vi "Frog ear specs.vi"(0 "ear folder path":path=path "/AJH L1.226B Q800/LabVIEW 3.0.1/Data/MEB/94/09/06.01/Ear 1") -> ()   [LabVIEW 2010]
panel:
  in  "time BPN' thaw":string="Time of BPN' thawing: XX"
  in  "OM removal":string="Ease of OM removal: XX"
  in  "Rating criterion":string="NOTE: Answer relative questions with a 1-10 scale (1 worst case; 10 ideal)"
  in  "mass":string="Mass (g): XX - XX"
  in  "Length (mm)":string="Length (mm): XX (mouth tip to extended leg) - XX"
  in  "Sex":string="Sex: XX"
  in  "Other comments about preparation:":string="Other comments about preparation: none"
  in  "Other comments about organ mounting:":string="Other comments about organ mounting: none"
  in  "Other comments about BPN'ing:":string="Other comments about BPN'ing: none"
  in  "Other comments about organ attainment:":string="Other comments about organ attainment: none"
  in  "Seeming approachability to kcbs:":string="Seeming approachability to kcbs: XX"
  in  "Perpendicularity of hb stereocilia:":string="Perpendicularity of hb stereocilia:  XX"
  in  "Amount of goo & crystals around hbs:":string="Amount of goo & crystals around hbs: XX"
  in  "Hair bundles' general condition:":string="Hair bundles' general condition: XX"
  in  "Amount of any further NSE desintegration:":string="Amount of any further NSE desintegration: XX"
  in  "Closeness of nerve cut to macula:":string="Closeness of nerve cut to macula: XX"
  in  "Flatness of macula as judged from dissection scope:":string="Macular flatness: XX"
  in  "Amount of sticking of organ to Pasteur pipette while transfereing organ from BPN' dish to solution dish to experimental chamber:":string="Amount of sticking of organ to Pasteur pipette while transfereing organ from BPN' dish to solution dish to chamber: XX"
  in  "# pins used to mount organ:":string="# pins used to mount organ: XX"
  in  "Amount of NSE desintegrationduring BPN'ing:":string="Amount of NSE degradation during BPN'ing: XX"
  in  "Organ BPN'ing facing:":string="Organ BPN'ing facing: XX"
  in  "Amount of sticking of organ to Pasteur pipette while transfereing organ to BPN' dish:":string="Amount of sticking of organ to Pasteur pipette while transfereing organ to BPN' dish: XX"
  in  "OM peeling?":string="Portion of OM peeled away: XX"
  in  "Crystals over OM?":string="Amount of leftover crystals atop OM: XX"
  in  "Leftover NSE goo?":string="Amount of leftover NSE goo: XX"
  in  "Any mechanical trauma to ear during organ dissection from inner ear?":string="Mechanical trauma to ear during organ dissection from inner ear: XX"
  in  "Goo removal easy?":string="Ease of goo removal: XX"
  in  "Inner ear removal from frog head through a meniscus?":string="Inner ear removal from frog head through a meniscus (T/F): XX"
  in  "Mechanical trauma to organ during inner ear dissection from animal:":string="Mechanical trauma to organ during inner ear dissection from animal: XX"
  in  "Saline oxygenation time (min)":string="Solution oxygenation time: XX"
  in  "OK; save & end":bool
  in  "BPN' time (min)":string="BPN' time (min): XX"
  in  "[BPN'] (mg/ml)":string="[BPN'] (mg/ml): XX"
  in  "Dissection solution":string="Dissection solution: Standard saline"
  in  "Organ":string="Organ: Sacculus"
  in  "Animal species":string="Species: Rana catesbeiana"
  in  "Animal death time":string="Time of death: XX"
  # "HARD SPECS:"
  # "SOLUTIONS:"
  # "ORGAN ATTAINMENT:"
  # "BPN'ing:"
  # "ORGAN MOUNTING:"
  # "CELLULAR (as judged under experimental scope):"
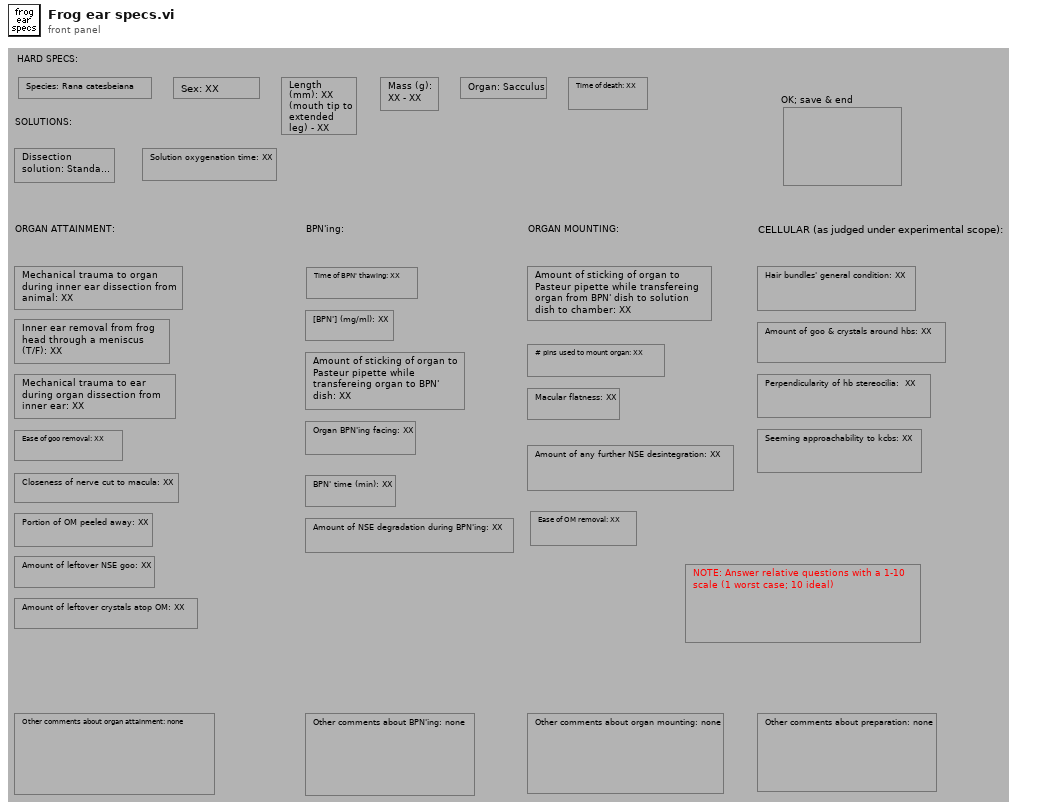
[diagram p1: front panel]
types:
  T1 = cluster{i32, i32, i32, i32, i32, i32, i32, i32, i32}
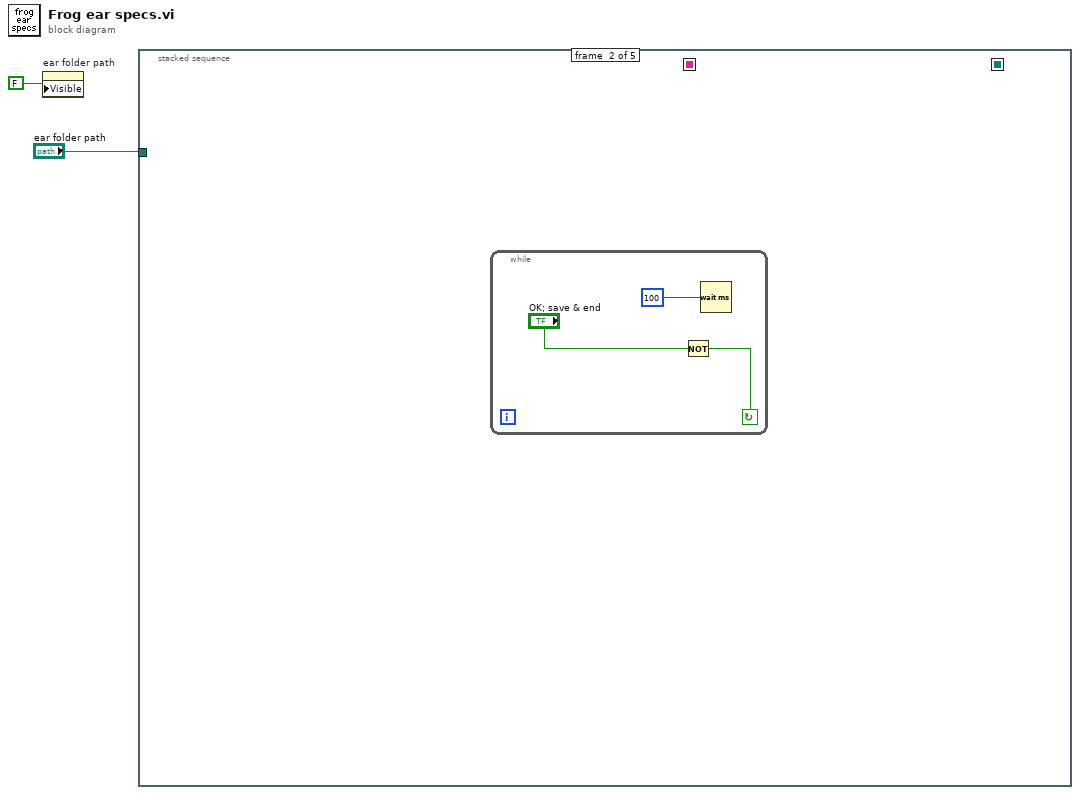
[diagram p0: block diagram]
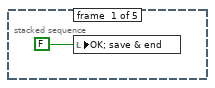
[diagram p2: hidden frame]
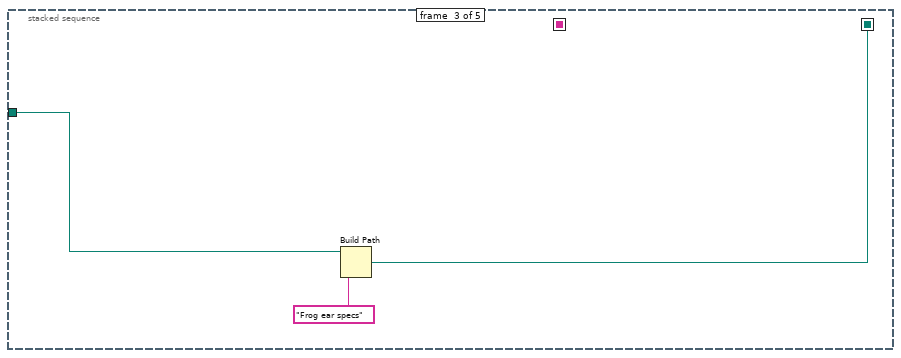
[diagram p3: hidden frame]
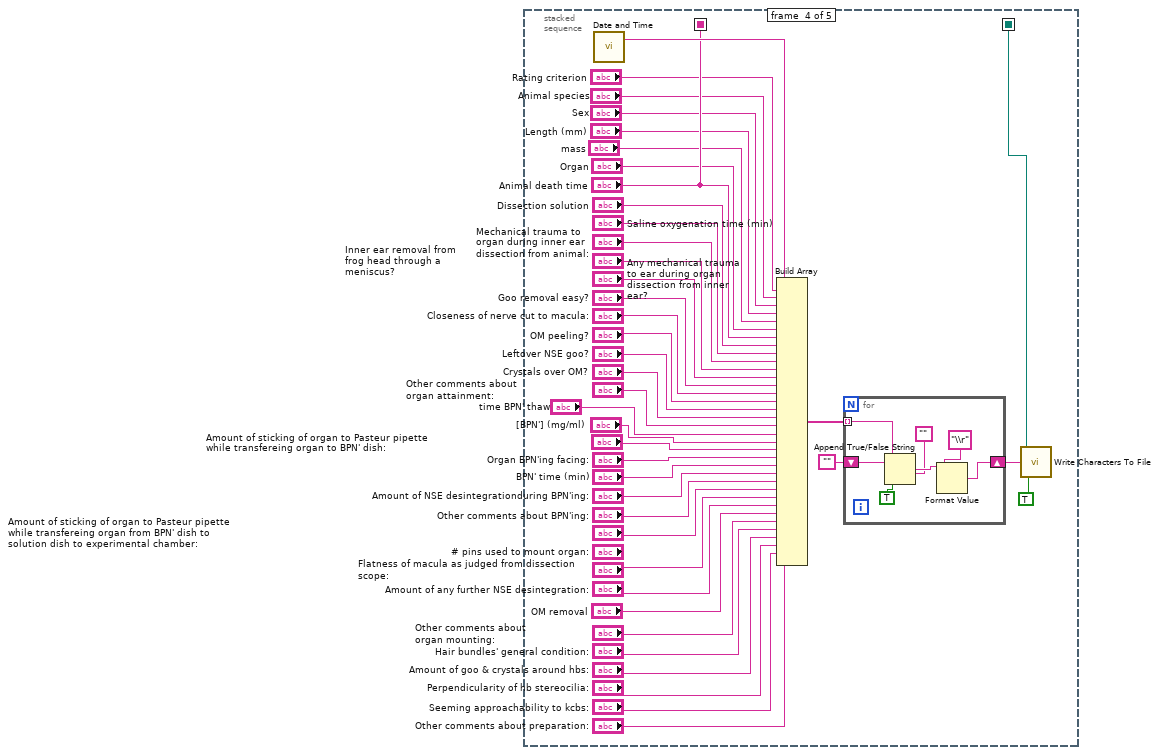
[diagram p4: hidden frame]
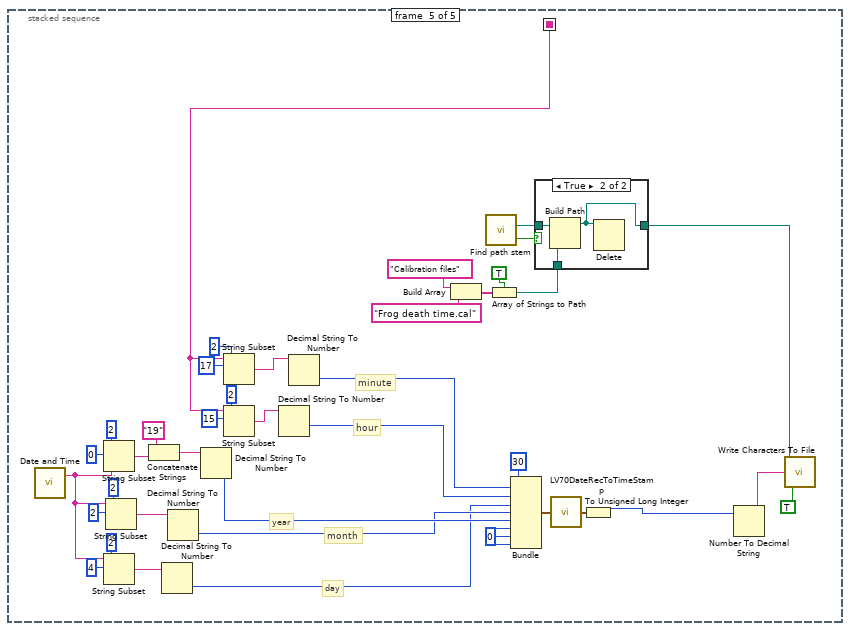
[diagram p5: hidden frame]
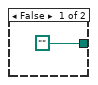
[diagram p6: hidden frame]
diagram:
  n1 = property on="ear folder path" class="Path"("Visible"=FALSE) -> ()  [unwired: 2 in, 2 out]
  n2 = stacked-sequence {
    seq-local: [_ _ w7 _ _] -> [_ _ _ w46 _]
    seq-local: [_ _ _ "Animal death time" _] -> [_ _ _ _ w61]
    tunnel: "ear folder path" -> [_ _ w8 _ _]
    frame #0 {
      n3 = local write "OK; save & end"(FALSE) -> ()
    }
    frame #1 {
      n4 = while {
        stop <- w6 continue-if-true
        n5 = Not(x="OK; save & end") -> (.not. x?=w6:bool)
        n6 = Wait (ms)(milliseconds to wait=100) -> ()  [unwired: 1 out]
      }
    }
    frame #2 {
      n7 = Build Path(base path=w8, name or relative path="Frog ear specs") -> (appended path=w7:path)
    }
    frame #3 {
      n8 = call "Date and Time.vi"() -> ("Date string."=w45:string)  [unwired: 1 out]
      n9 = Build Array(w45, "Rating criterion", "Animal species", "Sex", "Length (mm)", "mass", "Organ", "Animal death time", "Dissection solution", "Saline oxygenation time (min)", "Mechanical trauma to organ during inner ear dissection from animal:", "Inner ear removal from frog head through a meniscus?", "Any mechanical trauma to ear during organ dissection from inner ear?", "Goo removal easy?", "Closeness of nerve cut to macula:", "OM peeling?", "Leftover NSE goo?", "Crystals over OM?", "Other comments about organ attainment:", "time BPN' thaw", "[BPN'] (mg/ml)", "Amount of sticking of organ to Pasteur pipette while transfereing organ to BPN' dish:", "Organ BPN'ing facing:", "BPN' time (min)", "Amount of NSE desintegrationduring BPN'ing:", "Other comments about BPN'ing:", "Amount of sticking of organ to Pasteur pipette while transfereing organ from BPN' dish to solution dish to experimental chamber:", "Flatness of macula as judged from dissection scope:", "Amount of any further NSE desintegration:", "OM removal", "Other comments about organ mounting:", "Hair bundles' general condition:", "Amount of goo & crystals around hbs:", "Perpendicularity of hb stereocilia:", "Seeming approachability to kcbs:", "Other comments about preparation:") -> (w48:string[])
      n10 = for {
        tunnel: w48 -> [w55] mode=indexing
        shift-right: [w52] -> w50
        shift-left: "" -> [w56]
        n11 = Append True/False String(1:TRUE, 2:"", 3:w55, 4:w56) -> (0:w53:string)
        n12 = Format Value(string ("")=w53, format string="\\r") -> (output string=w52:string)  [unwired: 1 out]
      }
      n13 = call <vilib>:"Write Characters To File.vi"("append to file? (new file:F)"=TRUE, "character string"=w50, "file path (dialog if empty)"=w46) -> ()  [unwired: 3 out]
    }
    frame #4 {
      w87 = 0
      # "day"
      # "month"
      # "year"
      # "hour"
      # "minute"
      n14 = call "Date and Time.vi"() -> ("Date string."=w71:string)  [unwired: 1 out]
      n15 = String Subset(string=w71, offset (0)=0, length (rest)=2) -> (substring=w80:string)
      n16 = String Subset(string=w71, offset (0)=4, length (rest)=2) -> (substring=w70:string)
      n17 = String Subset(string=w71, offset (0)=2, length (rest)=2) -> (substring=w75:string)
      n18 = Concatenate Strings("19", w80) -> (w79:string)
      n19 = Decimal String To Number(string=w70) -> (number=w69:i32)  [unwired: 3 out]
      n20 = Decimal String To Number(string=w75) -> (number=w74:i32)  [unwired: 3 out]
      n21 = Decimal String To Number(string=w79) -> (number=w78:i32)  [unwired: 3 out]
      n22 = String Subset(string=w61, offset (0)=17, length (rest)=2) -> (substring=w93:string)
      n23 = String Subset(string=w61, offset (0)=15, length (rest)=2) -> (substring=w91:string)
      n24 = Decimal String To Number(string=w91) -> (number=w88:i32)  [unwired: 3 out]
      n25 = Decimal String To Number(string=w93) -> (number=w92:i32)  [unwired: 3 out]
      n26 = Build Array("Calibration files", "Frog death time.cal") -> (w65:string[])
      n27 = call "Find path stem.vi"() -> ("PASS/FAIL"=w63:bool, "Path stem."=w64:path)
      n28 = Array of Strings to Path(0:w65, 1:TRUE) -> (2:w62:path)
      n29 = Bundle(30, w92, w88, w69, w74, w78, w87, w87, w87) -> (w95:T1)  [unwired: 1 out]
      n30 = case shown="True" w63 {
        tunnel: w64 -> [_ w100]
        tunnel: w62 -> [_ w99]
        tunnel: [path "" w98] -> w60
        frame False {
        }
        frame True {
          n31 = Build Path(base path=w100, name or relative path=w99) -> (appended path=w98:path)
          n32 = Delete(path (use dialog)=w98) -> ()  [unwired: 1 in, 6 out]
        }
      }
      n33 = call <vilib>:"LV70DateRecToTimeStamp.vi"("date time rec"=w95) -> ("Time Stamp"=w58:timestamp)
      n34 = To Unsigned Long Integer(number=w58) -> (unsigned 32bit integer=w59:u32)
      n35 = Number To Decimal String(number=w59) -> (decimal integer string=w96:string)  [unwired: 1 out]
      n36 = call <vilib>:"Write Characters To File.vi"("append to file? (new file:F)"=TRUE, "character string"=w96, "file path (dialog if empty)"=w60) -> ()  [unwired: 3 out]
    }
  }
